vi "QueueDispose.vi"(8 "error in (no error)":errorcluster, 11 "Execute":refnum<class "Execute.lvclass">) -> (0 "error out":errorcluster, 3 "Execute":refnum<class "Execute.lvclass">)   [LabVIEW 2018, in "QMH_Class.lvlib" / "TestManager.lvlib" / "Execute.lvclass"]
uses:
  Execute.lvclass
  Execute.lvclass/Execute.ctl
  Message_class/InterfaceMessage/Interface Message.lvclass
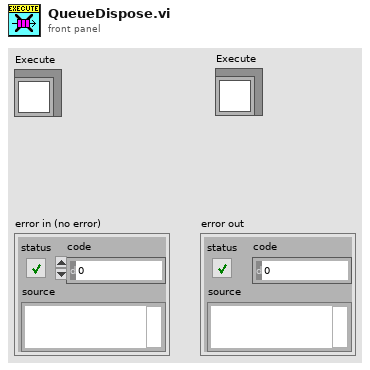
[diagram p1: front panel]
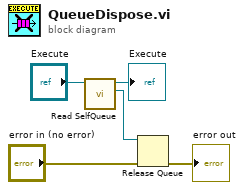
[diagram p0: block diagram]
diagram:
  n1 = call "Read SelfQueue.vi"("Execute"="Execute") -> ("SelfQueue"=w4:refnum<queue>, "Execute"=→"Execute":refnum<class "Execute.lvclass">)  [unwired: 8 in, 1 out]
  n2 = Release Queue(queue=w4, error in (no error)="error in (no error)") -> (error out=→"error out":errorcluster)  [unwired: 1 in, 2 out]
